vi "Write auto_.vi"(8 "error in (no error)":errorcluster, 10 "auto?":bool, 11 "Change Speaker Cycle Params in":refnum<class "Change Speaker Cycle Params.lvclass">) -> (0 "error out":errorcluster, 3 "Change Speaker Cycle Params out":refnum<class "Change Speaker Cycle Params.lvclass">)   [LabVIEW 2017, in "Change Speaker Cycle Params.lvclass"]
uses:
  Change Speaker Cycle Params.lvclass
  Change Speaker Cycle Params.lvclass/Change Speaker Cycle Params.ctl
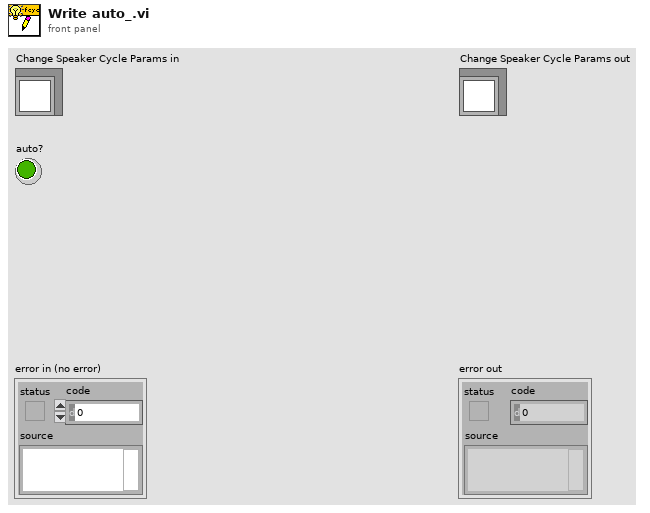
[diagram p1: front panel]
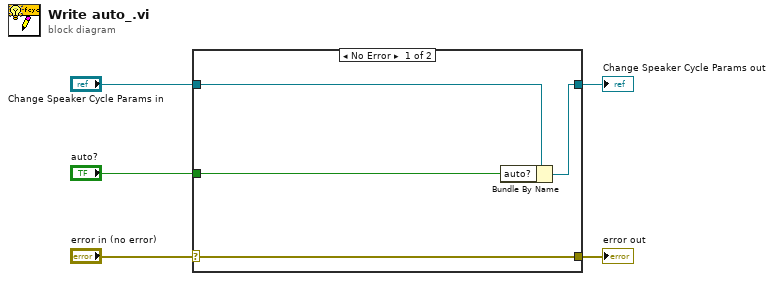
[diagram p0: block diagram]
diagram:
  n1 = case shown="No Error" "error in (no error)" {
    selector: "error in (no error)" -> [w9 w10]
    tunnel: [w9 w10] -> w4
    tunnel: [w7 w11] -> w2
    tunnel: "Change Speaker Cycle Params in" -> [w8 w11]
    tunnel: "auto?" -> [w6 _]
    frame No Error {
      n2 = Bundle By Name(cluster=w8, "auto?"=w6) -> (w7:refnum<class "Change Speaker Cycle Params.lvclass">)
    }
    frame Error {
    }
  }
  "error out" <- w4
  "Change Speaker Cycle Params out" <- w2
